vi "Test.Maui 2.0.Initialize.Scarce.Rings.Ring 2.vi"(8 "error in":errorcluster) -> (0 "error out":errorcluster)   [LabVIEW 2020]
uses:
  Maui 2.0/Maui 2.0.lvclass
  C:/Program Files (x86)/National Instruments/LabVIEW 2020/vi.lib/JKI/JKI SMO/SMO/SMO.lvclass
  Helper/Test Helper 1/Test Helper 1.lvclass
  <vilib>/addons/_JKI Toolkits/Caraya/classes/Assert/Assert Equal Value_Variant.vi
  <vilib>/JKI/JKI SMO/SMO/SMO.lvclass
  <vilib>/addons/_JKI Toolkits/Caraya/classes/Assert/Assert.lvclass
  <vilib>/addons/_JKI Toolkits/Caraya/classes/Test/Test.lvclass
panel:
  in  "Ring 2":u16(ring) items=["Test Helper 1", "None"]
  in  "Ring":u16(ring) items=["Test Helper 1", "None"]
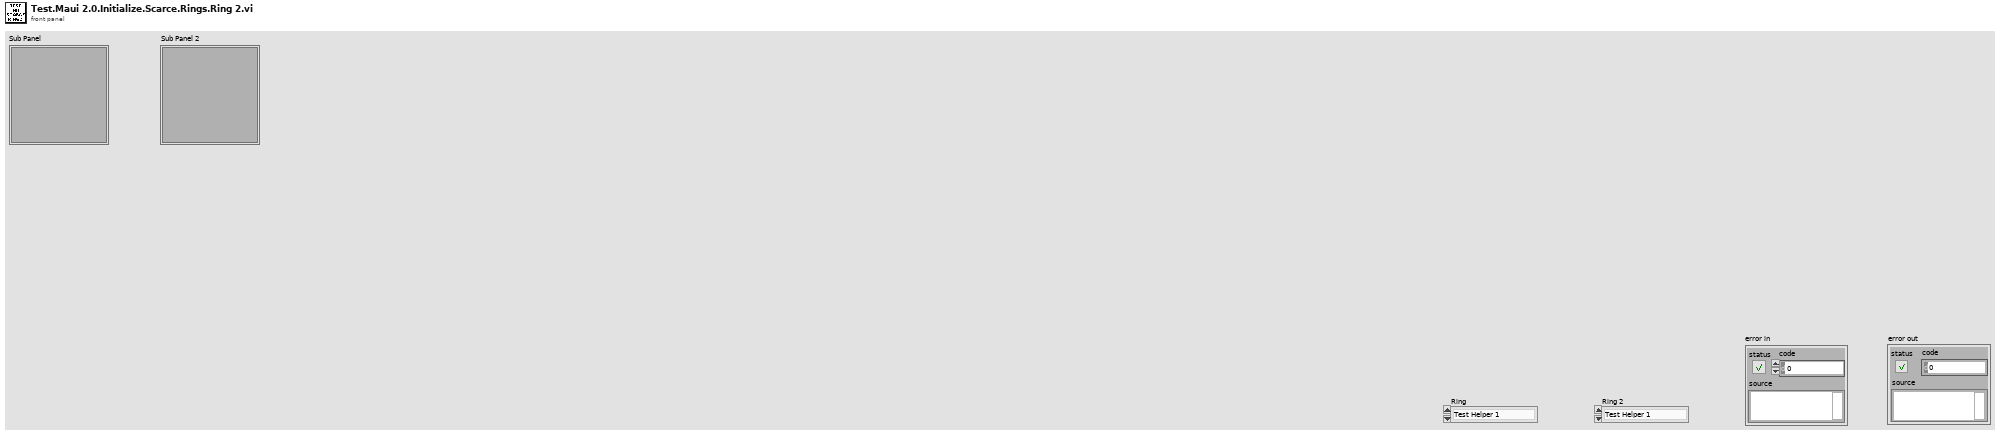
[diagram p1: front panel]
types:
  T1 = cluster{"Ring":refnum<vi>, "Sub Panel":refnum<vi>}
  T2 = cluster{"Ring 2":refnum<vi>, "Sub Panel 2":refnum<vi>}
  T3 = cluster{"Ring 2":refnum<vi>, "Sub Panel 2":refnum<vi>}[]
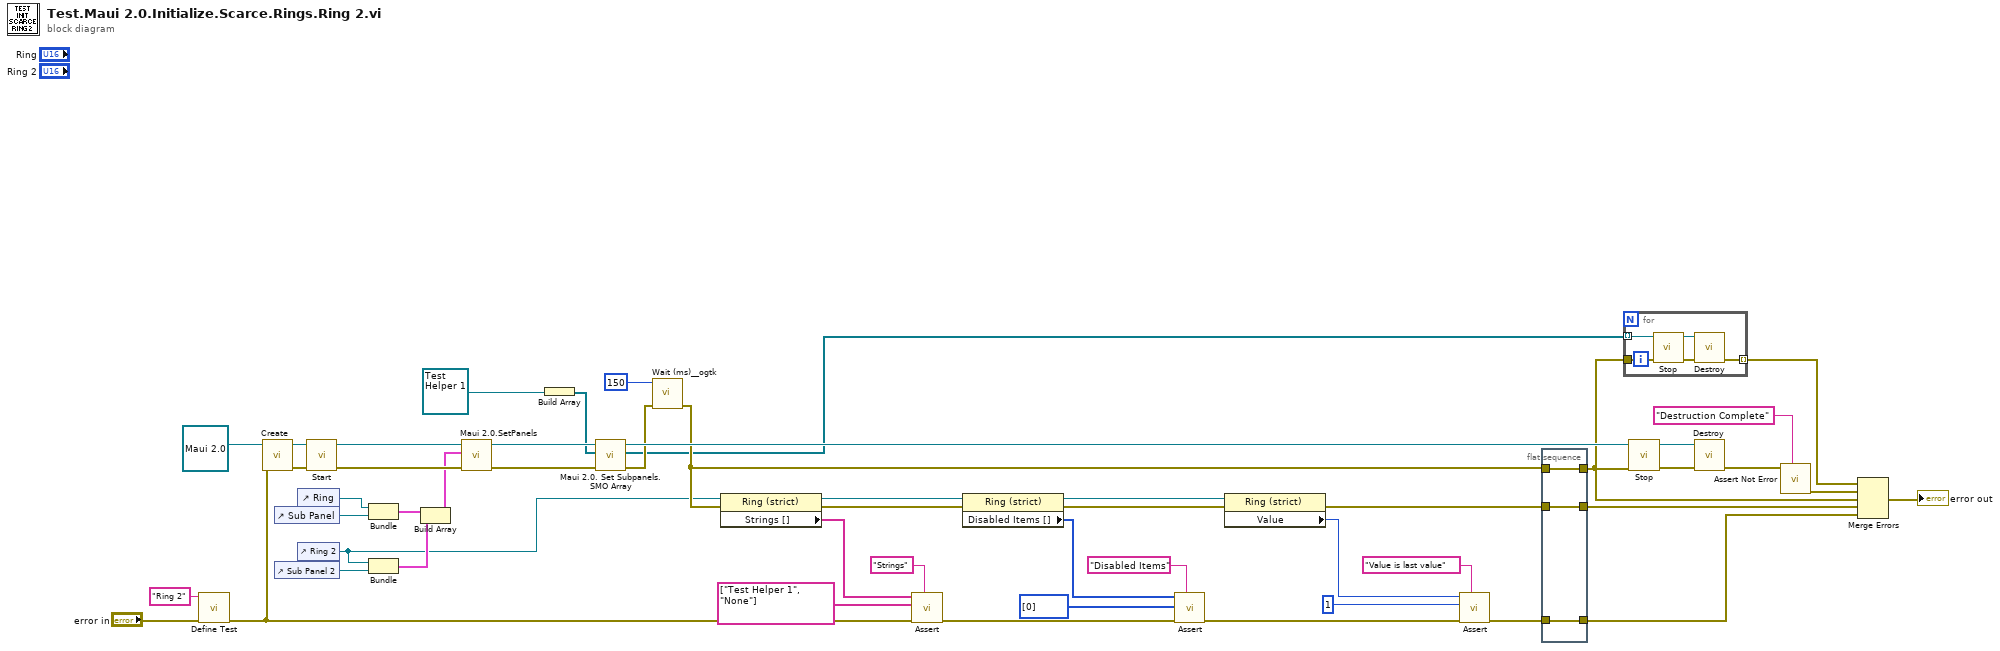
[diagram p0: block diagram]
diagram:
  n1 = call <vilib>:"Define Test.vi"("error in (no error)"="error in", "Label (VI Title)"="Ring 2") -> ("error out"=w27:errorcluster)  [unwired: 9 in]
  n2 = call <vilib>:"Create.vi"("error in (no error)"=w27, "SMO"=refnum<class "Maui 2.0.lvclass"> refnum ("Maui 2.0 in")) -> ("error out"=w51:errorcluster, "SMO out"=w44:refnum<class "Maui 2.0.lvclass">)  [unwired: 7 in, 1 out]
  n3 = control-ref of="Sub Panel"() -> (w48:refnum<vi>)
  n4 = control-ref of="Sub Panel 2"() -> (w47:refnum<vi>)
  n5 = control-ref of="Ring"() -> (w37:refnum<vi>)
  n6 = control-ref of="Ring 2"() -> (w2:refnum<vi>)
  n7 = call <vilib>:"Start.vi"("error in (no error)"=w51, "SMO"=w44) -> ("error out"=w50:errorcluster, "SMO out"=w42:refnum<class "Maui 2.0.lvclass">)  [unwired: 8 in]
  n8 = Bundle("Ring"=w37, "Sub Panel"=w48) -> (w46:T1)  [unwired: 1 in]
  n9 = Bundle("Ring 2"=w2, "Sub Panel 2"=w47) -> (w45:T2)  [unwired: 1 in]
  n10 = Build Array(w46, w45) -> (w38:T3)
  n11 = call "Maui 2.0.SetPanels.vi"("error in (no error)"=w50, "Set Panels"=w38, "Maui 2.0"=w42) -> ("error out"=w49:errorcluster, "Maui 2.0 out"=w41:refnum<class "Maui 2.0.lvclass">)  [unwired: 7 in]
  n12 = Build Array(refnum<class "Test Helper 1.lvclass"> refnum ("Test Helper 1.lvclass")) -> (w39:refnum<class "Test Helper 1.lvclass">[])
  n13 = call-dynamic "Maui 2.0. Set Subpanels.SMO Array.vi"("error in (no error)"=w49, "Subpanels in"=w39, "Maui 2.0 in"=w41) -> ("error out"=w11:errorcluster, "Subpanels Out"=w8:refnum<class "SMO.lvclass">[], "Maui 2.0 out"=w21:refnum<class "Maui 2.0.lvclass">)  [unwired: 6 in]
  n14 = call <userlib>:"Wait (ms)__ogtk.vi"("error in (no error)"=w11, "milliseconds to wait"=u32 150) -> ("error out"=w10:errorcluster)  [unwired: 8 in, 1 out]
  n15 = property on="Property Node" class="Ring (strict)"(reference=w2, error in=w10) -> (reference out=w31:refnum<vi>, error out=w24:errorcluster, "Strings []"=w35:string[])
  n16 = call-poly <vilib>:"Assert.vi"("Label"="Strings", "error in (no error)"=w27, "Y"=string[] ["Test Helper 1", "None"], "X"=w35) -> ("error out"=w25:errorcluster)  [unwired: 7 in]
  n17 = property on="Property Node" class="Ring (strict)"(reference=w31, error in=w24) -> (reference out=w29:refnum<vi>, error out=w23:errorcluster, "Disabled Items []"=w5:i32[])
  n18 = call-poly <vilib>:"Assert.vi"("Label"="Disabled Items", "error in (no error)"=w25, "Y"=i32[] [0] ("Disabled Items []"), "X"=w5) -> ("error out"=w26:errorcluster)  [unwired: 7 in]
  n19 = property on="Property Node" class="Ring (strict)"(reference=w29, error in=w23) -> (error out=w15:errorcluster, "Value"=w22:u16)  [unwired: 1 out]
  n20 = call-poly <vilib>:"Assert.vi"("Label"="Value is last value", "error in (no error)"=w26, "Y"=u16 1 ("Value"), "X"=w22) -> ("error out"=w14:errorcluster)  [unwired: 7 in]
  n21 = flat-sequence {
    tunnel: w10 -> [w54]
    tunnel: w15 -> [w53]
    tunnel: w14 -> [w52]
    tunnel: [w54] -> w6
    tunnel: [w53] -> w13
    tunnel: [w52] -> w12
    frame #0 {
    }
  }
  n22 = for {
    tunnel: w8 -> [w58] mode=indexing
    tunnel: w6 -> [w57]
    tunnel: [w55] -> w7 mode=indexing
    n23 = call <vilib>:"Stop.vi"("error in (no error)"=w57, "SMO"=w58) -> ("error out"=w56:errorcluster, "SMO out"=w59:refnum<class "SMO.lvclass">)  [unwired: 8 in]
    n24 = call <vilib>:"Destroy.vi"("error in (no error)"=w56, "SMO"=w59) -> ("error out"=w55:errorcluster)  [unwired: 9 in]
  }
  n25 = call <vilib>:"Stop.vi"("error in (no error)"=w6, "SMO"=w21) -> ("error out"=w19:errorcluster, "SMO out"=w20:refnum<class "Maui 2.0.lvclass">)  [unwired: 8 in]
  n26 = call <vilib>:"Destroy.vi"("error in (no error)"=w19, "SMO"=w20) -> ("error out"=w18:errorcluster)  [unwired: 9 in]
  n27 = call <vilib>:"Assert Not Error.vi"("Label"="Destruction Complete", "Not Error?"=w18) -> ("error out"=w16:errorcluster)  [unwired: 9 in]
  n28 = Merge Errors(w7, w16, w6, w13, w12) -> (→"error out":errorcluster)
